vi "Supply_SetVolts.vi"(8 "error in (no error)":errorcluster, 9 "Command string":string, 10 "Current IN [V]":dbl, 11 "KE2410 in":refnum<class "R_Metal_KE2410.lvclass">) -> (0 "error out":errorcluster, 2 "Compliance exceeded?":bool, 3 "KE2410 out":refnum<class "R_Metal_KE2410.lvclass">)   [LabVIEW 2019, in "R_Metal_KE2410.lvclass"]
uses:
  R_Metal_KE2410.lvclass
  InstrumentSetup.vi
  SupplyControl.lvclass
  InstrControl.lvclass
panel:
  out "Command sent":string
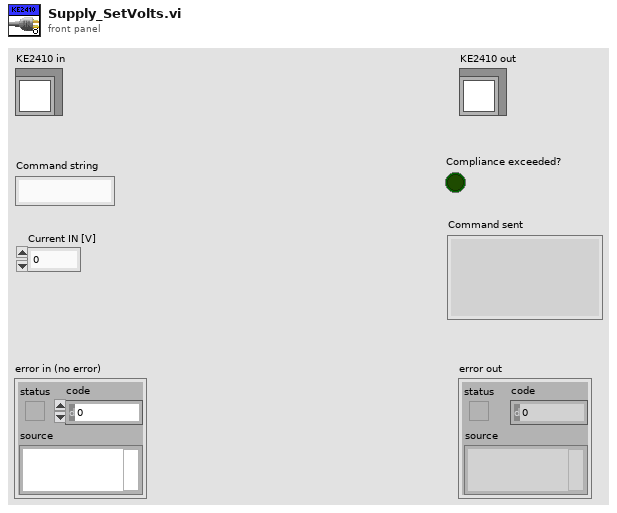
[diagram p1: front panel]
types:
  T1 = cluster{"Voltage Limit":sgl, "R_Metal_KE2410":refnum<class "R_Metal_KE2410.lvclass">}
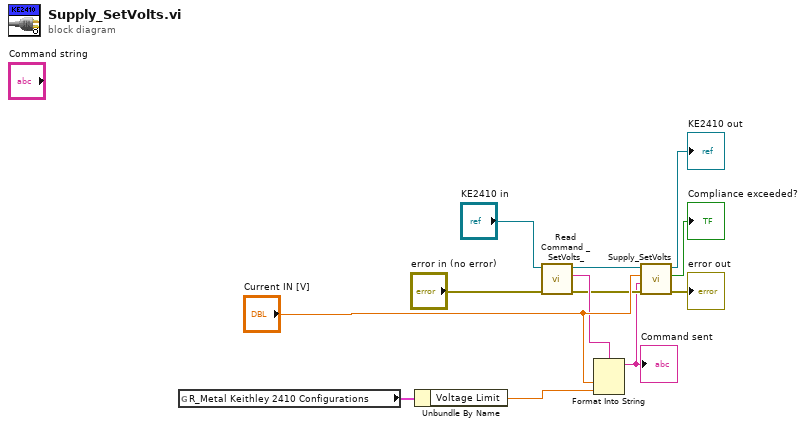
[diagram p0: block diagram]
diagram:
  n1 = global read "InstrumentSetup.vi" "R_Metal Keithley 2410 Configurations"() -> (w9:T1)
  n2 = Unbundle By Name(w9) -> ("Voltage Limit"=w1:sgl)
  n3 = call-dynamic "Read Command _SetVolts_.vi"("error in (no error)"="error in (no error)", "SupplyControl in"="KE2410 in") -> ("error out"=w4:errorcluster, "Command \"SetVolts\""=w5:string, "SupplyControl out"=w3:refnum<class "R_Metal_KE2410.lvclass">)  [unwired: 7 in]
  n4 = Format Into String(format string=w5, "Current IN [V]", w1) -> (resulting string=w2:string)  [unwired: 2 in, 1 out]
  "Command sent" <- w2
  n5 = call-parent "Supply_SetVolts.vi"("error in (no error)"=w4, "Command string"=w2, "Volts IN [V]"="Current IN [V]", "SupplyControl in"=w3) -> ("error out"=→"error out":errorcluster, "Compliance exceeded?"=→"Compliance exceeded?":bool, "SupplyControl out"=→"KE2410 out":refnum<class "R_Metal_KE2410.lvclass">)  [unwired: 5 in]
